vi "integrated_prac_merge1.vi"() -> ()   [LabVIEW 2014]
uses:
  <instrlib>/KD Scientific 2XX Series/KD Scientific 2XX Series.lvlib
panel:
  out "Units":string
  out "Delivered Volume":dbl
  in  "stop":bool
  out "Status":T1
  in  "Flow Rate (5)":dbl=5.0
  in  "Units (0: milliliters)":u16(ring) items=["milliliters (ml)", "microliters (ul)"]
  in  "Volume (100)":dbl=100.0
  in  "Diameter (8.75 mm)":dbl=8.75
  in  "Mode (infuse)":u16(ring) items=["Infuse", "Withdraw", "Infuse-Withdraw", "Withdraw-Infuse", "Continuous"]
  in  "Address (0)":i32
  in  "error in (no error)":errorcluster
  in  "Baud Rate (9600)":u32(ring)=9600 items=["300"=300, "1200"=1200, "2400"=2400, "4800"=4800, "9600"=9600]
  in  "VISA resource name":refnum<visa-resource-name>
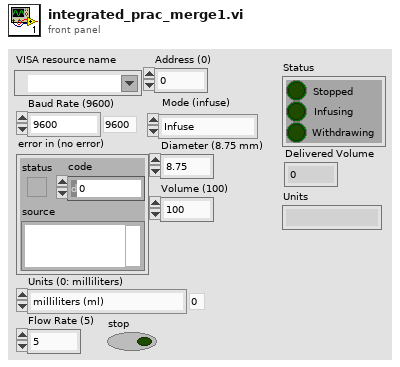
[diagram p1: front panel]
types:
  T1 = cluster{"Stopped":bool, "Infusing":bool, "Withdrawing":bool}
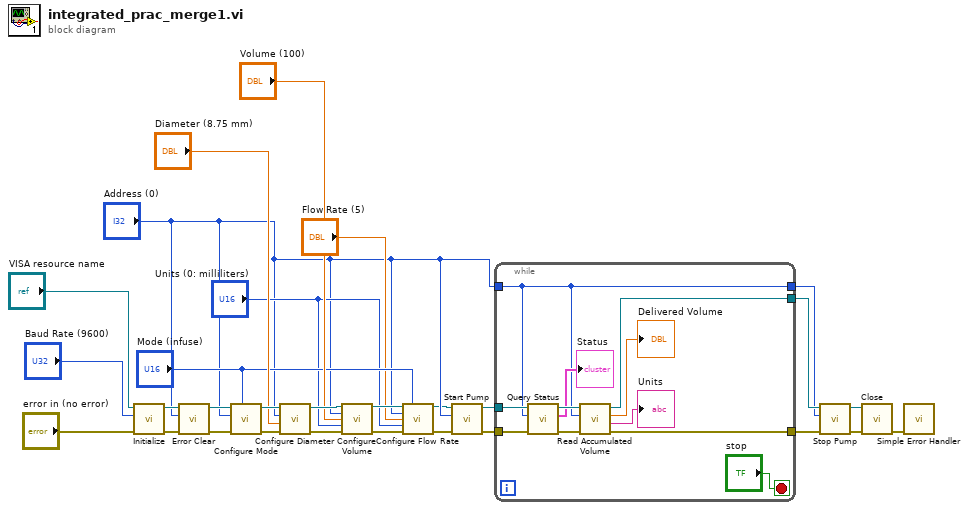
[diagram p0: block diagram]
diagram:
  n1 = call <instrlib>:"Initialize.vi"("error in (no error)"="error in (no error)", "Baud Rate (9600)"="Baud Rate (9600)", "VISA resource name"="VISA resource name") -> ("error out"=w25:errorcluster, "VISA resource name out"=w26:refnum<visa-resource-name>)  [unwired: 7 in]
  n2 = call <instrlib>:"Error Clear.vi"("error in (no error)"=w25, "Address (0)"="Address (0)", "VISA resource name"=w26) -> ("error out"=w23:errorcluster, "VISA resource name out"=w24:refnum<visa-resource-name>)  [unwired: 6 in, 1 out]
  n3 = call <instrlib>:"Configure Mode.vi"("Mode (infuse)"="Mode (infuse)", "error in (no error)"=w23, "Address (0)"="Address (0)", "VISA resource name"=w24) -> ("error out"=w13:errorcluster, "VISA resource name out"=w14:refnum<visa-resource-name>)  [unwired: 6 in]
  n4 = call <instrlib>:"Configure Diameter.vi"("error in (no error)"=w13, "Diameter (8.75 mm)"="Diameter (8.75 mm)", "Address (0)"="Address (0)", "VISA resource name"=w14) -> ("error out"=w10:errorcluster, "VISA resource name out"=w11:refnum<visa-resource-name>)  [unwired: 6 in]
  n5 = call <instrlib>:"Configure Volume.vi"("VISA resource name"=w11, "Address (0)"="Address (0)", "Volume (100)"="Volume (100)", "Units (0: milliliters)"="Units (0: milliliters)", "error in (no error)"=w10) -> ("VISA resource name out"=w8:refnum<visa-resource-name>, "error out"=w7:errorcluster)  [unwired: 9 in]
  n6 = call <instrlib>:"Configure Flow Rate.vi"("VISA resource name"=w8, "Mode (infuse)"="Mode (infuse)", "Address (0)"="Address (0)", "Flow Rate (5)"="Flow Rate (5)", "Units (0: milliliters per minute)"="Units (0: milliliters)", "error in (no error)"=w7) -> ("VISA resource name out"=w2:refnum<visa-resource-name>, "error out"=w1:errorcluster)  [unwired: 8 in]
  n7 = call <instrlib>:"Start Pump.vi"("error in (no error)"=w1, "Address (0)"="Address (0)", "VISA resource name"=w2) -> ("error out"=w21:errorcluster, "VISA resource name out"=w22:refnum<visa-resource-name>)  [unwired: 7 in]
  n8 = while {
    tunnel: w22 -> [w40]
    tunnel: w21 -> [w39]
    tunnel: "Address (0)" -> [w31]
    tunnel: [w33] -> w20
    tunnel: [w32] -> w19
    tunnel: [w31] -> w18
    stop <- "stop" stop-if-true
    n9 = call <instrlib>:"Query Status.vi"("error in (no error)"=w39, "Address (0)"=w31, "VISA resource name"=w40) -> ("error out"=w37:errorcluster, "Status"=→"Status":T1, "VISA resource name out"=w38:refnum<visa-resource-name>)  [unwired: 6 in]
    n10 = call <instrlib>:"Read Accumulated Volume.vi"("error in (no error)"=w37, "Address (0)"=w31, "VISA resource name"=w38) -> ("error out"=w32:errorcluster, "Units"=→"Units":string, "Delivered Volume"=→"Delivered Volume":dbl, "VISA resource name out"=w33:refnum<visa-resource-name>)  [unwired: 5 in]
  }
  n11 = call <instrlib>:"Stop Pump.vi"("error in (no error)"=w19, "Address (0)"=w18, "VISA resource name"=w20) -> ("error out"=w16:errorcluster, "VISA resource name out"=w17:refnum<visa-resource-name>)  [unwired: 7 in]
  n12 = call <instrlib>:"Close.vi"("error in (no error)"=w16, "VISA resource name"=w17) -> ("error out"=w15:errorcluster)  [unwired: 9 in]
  n13 = call <vilib>:"Simple Error Handler.vi"("error in (no error)"=w15) -> ()  [unwired: 4 in, 5 out]
